vi "IMAQController.SubCameraFromCameraList.vi"(0 "i ref in":refnum<vi>, 2 "CS Camera Name":string, 5 "error in (no error)":errorcluster) -> (14 "i ref out":refnum<vi>, 16 "actItem Number":i32[](array[numeric]), 17 "Item Names":string[][](array[string]), 19 "error out":errorcluster)   [LabVIEW 2014, in "IMAQController.lvlib"]
uses:
  IMAQController.lvlib
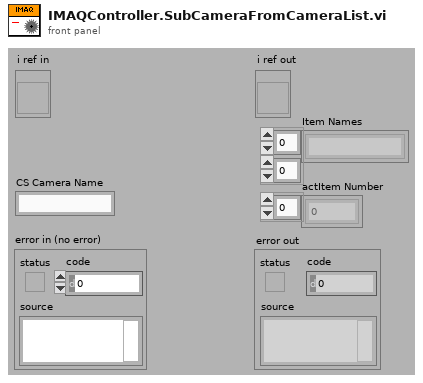
[diagram p1: front panel]
types:
  T1 = typedef "IMAQController.lvlib/IMAQController.i attribute.ctl" = cluster{"ImageTakenID":i32, "actSequencer":string, "actScanner":string, "CameraTriggerID":i32, "activatedCameras":cluster{"Name":string, "Camera Type":string, "Acquisition Mode":u32, "JPEG Mode?":bool, "Acquisition Delay":dbl, "Save Images?":bool, "Center Coordinates":T2, "PixelPermm":cluster{"Horizontal":dbl, "Vertical":dbl}, "Rotation":dbl, "Mirror Mode":u32, "PixelCoordinates":cluster{"1":cluster{"Horizontal":i32, "Vertical":i32}, "2":cluster{"Horizontal":i32, "Vertical":i32}, "3":cluster{"Horizontal":i32, "Vertical":i32}, "4":cluster{"Horizontal":i32, "Vertical":i32}}, "RWCoordinates":cluster{"1":cluster{"Horizontal":dbl, "Vertical":dbl}, "2":cluster{"Horizontal":dbl, "Vertical":dbl}, "3":cluster{"Horizontal":dbl, "Vertical":dbl}, "4":cluster{"Horizontal":dbl, "Vertical":dbl}}, "HorizScaling":dbl, "VertScaling":dbl}[], "Ini C-Array":string[], "actCamera":string, "activeCamera":cluster{"Name":string, "Camera Type":string, "Aqcuisation Mode":enum32{"Internal Trigger", "Scan", "free Running", "External Trigger"}, "JPEG Mode?":bool, "Acquisition Delay":dbl, "Save Images?":bool, "Center Coordinates":T2, "PixelPermm":cluster{"Horizontal":dbl, "Vertical":dbl}, "Rotation":dbl, "Mirror Mode":u32, "PixelCoordinates":cluster{"1":cluster{"Horizontal":i32, "Vertical":i32}, "2":cluster{"Horizontal":i32, "Vertical":i32}, "3":cluster{"Horizontal":i32, "Vertical":i32}, "4":cluster{"Horizontal":i32, "Vertical":i32}}, "RWCoordinates":cluster{"1":cluster{"Horizontal":dbl, "Vertical":dbl}, "2":cluster{"Horizontal":dbl, "Vertical":dbl}, "3":cluster{"Horizontal":dbl, "Vertical":dbl}, "4":cluster{"Horizontal":dbl, "Vertical":dbl}}, "HorizScaling":dbl, "VertScaling":dbl}, "BilderMittelungen":u8, "OldPicture":dbl[][]}
  T2 = typedef "LVPoint32TypeDef.ctl" = cluster{"Horizontal":i32, "Vertical":i32}
  T3 = cluster{"Name":string, "Camera Type":string, "Acquisition Mode":u32, "JPEG Mode?":bool, "Acquisition Delay":dbl, "Save Images?":bool, "Center Coordinates":T2, "PixelPermm":cluster{"Horizontal":dbl, "Vertical":dbl}, "Rotation":dbl, "Mirror Mode":u32, "PixelCoordinates":cluster{"1":cluster{"Horizontal":i32, "Vertical":i32}, "2":cluster{"Horizontal":i32, "Vertical":i32}, "3":cluster{"Horizontal":i32, "Vertical":i32}, "4":cluster{"Horizontal":i32, "Vertical":i32}}, "RWCoordinates":cluster{"1":cluster{"Horizontal":dbl, "Vertical":dbl}, "2":cluster{"Horizontal":dbl, "Vertical":dbl}, "3":cluster{"Horizontal":dbl, "Vertical":dbl}, "4":cluster{"Horizontal":dbl, "Vertical":dbl}}, "HorizScaling":dbl, "VertScaling":dbl}[]
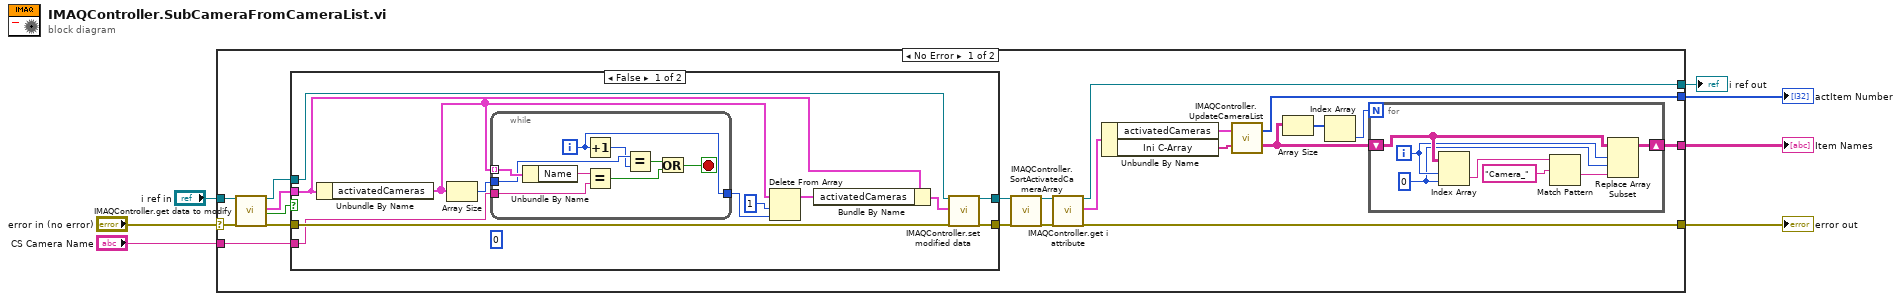
[diagram p0: block diagram]
diagram:
  n1 = case shown="No Error" "error in (no error)" {
    selector: "error in (no error)" -> [w25 w60]
    tunnel: [w16 w59] -> w7
    tunnel: [w15 w60] -> w6
    tunnel: "CS Camera Name" -> [w24 _]
    tunnel: "i ref in" -> [w26 w59]
    tunnel: [w9 _] -> w2
    tunnel: [w8 _] -> w1
    frame No Error {
      n2 = call "IMAQController.get data to modify.vi"("i ref in"=w26, "error in (no error)"=w25) -> ("i ref out"=w27:refnum<vi>, "i attribute"=w23:T1, "timed out"=w22:bool, "error out"=w28:errorcluster)  [unwired: 14 in]
      n3 = case shown="False" w22 {
        tunnel: w28 -> [w47 w57]
        tunnel: w27 -> [w46 w58]
        tunnel: [w45 w58] -> w21
        tunnel: [w44 w57] -> w20
        tunnel: w24 -> [w42 _]
        tunnel: w23 -> [w41 _]
        frame False {
          (unwired) 0 ("index")
          n4 = Unbundle By Name(w41) -> ("activatedCameras"=w39:T3)
          n5 = Array Size(array=w39) -> (size(s)=w43:i32)
          n6 = while {
            tunnel: w39 -> [w55] mode=indexing
            tunnel: w43 -> [w50]
            tunnel: w42 -> [w56]
            tunnel: [w48] -> w38
            i -> [w48]
            stop <- w53 stop-if-true
            n7 = Unbundle By Name(w55) -> ("Name"=w54:string)
            n8 = Increment(x=w48) -> (x+1=w49:i32)
            n9 = Equal?(x=w54, y=w56) -> (x = y?=w52:bool)
            n10 = Equal?(x=w50, y=w49) -> (x = y?=w51:bool)
            n11 = Or(x=w51, y=w52) -> (x .or. y?=w53:bool)
          }
          n12 = Delete From Array(array=w39, length=1, index=w38) -> (array with subset deleted=w36:T3)  [unwired: 1 out]
          n13 = Bundle By Name(cluster=w41, "activatedCameras"=w36) -> (w40:T1)
          n14 = call "IMAQController.set modified data.vi"("i ref in"=w46, "i attribute"=w40, "error in (no error)"=w47) -> ("i ref out"=w45:refnum<vi>, "error out"=w44:errorcluster)  [unwired: 15 in]
        }
        frame True {
        }
      }
      n15 = call "IMAQController.SortActivatedCameraArray.vi"("i ref in"=w21, "error in (no error)"=w20) -> ("i ref out"=w18:refnum<vi>, "error out"=w19:errorcluster)  [unwired: 16 in]
      n16 = call "IMAQController.get i attribute.vi"("i ref in"=w18, "error in (no error)"=w19) -> ("i ref out"=w16:refnum<vi>, "i attribute"=w17:T1, "error out"=w15:errorcluster)  [unwired: 15 in]
      n17 = Unbundle By Name(w17) -> ("activatedCameras"=w11:T3, "Ini C-Array"=w10:string[])
      n18 = call "IMAQController.UpdateCameraList.vi"("activatedCameras"=w11, "Detector.ini List Camera-Array"=w10) -> ("actItem Number"=w9:i32[], "Item Names"=w12:string[][])  [unwired: 16 in]
      n19 = Array Size(array=w12) -> (size(s)=w14:i32[])
      n20 = Index Array(array=w14) -> (element=w13:i32)  [unwired: 1 in]
      n21 = for {
        N: w13 -> [_]
        shift-right: [w29] -> w8
        shift-left: w12 -> [w33]
        i -> [w32]
        w31 = 0 ("disabled index (col)")
        n22 = Index Array(array=w33, index (row)=w32, index (col)=w31) -> (element=w35:string)
        n23 = Match Pattern(string=w35, regular expression="Camera_") -> (after substring=w30:string)  [unwired: 1 in, 3 out]
        n24 = Replace Array Subset(array=w33, new element=w30, index (row)=w32, index (col)=w31) -> (w29:string[][])
      }
    }
    frame Error {
    }
  }
  "i ref out" <- w7
  "error out" <- w6
  "actItem Number" <- w2
  "Item Names" <- w1
